vi "Close.vi"(8 "error in (no error)":errorcluster, 11 "Instrument.OxfordVRM in":refnum<class "Instrument.OxfordVRM.lvclass">) -> (0 "error out":errorcluster, 3 "Instrument.OxfordVRM out":refnum<class "Instrument.OxfordVRM.lvclass">)   [LabVIEW 2019, in "Instrument.OxfordVRM.lvclass"]
uses:
  Instrument.OxfordVRM.lvclass
  C:/Program Files (x86)/National Instruments/LabVIEW 2019/user.lib/LevyLab/Instrument Framework/Instrument/Instrument.lvclass
  <userlib>/LevyLab/Instrument Framework/Instrument Types/Cryostat/Instrument.Cryostat.lvclass
  <userlib>/LevyLab/Instrument Framework/Instrument/Instrument.lvclass
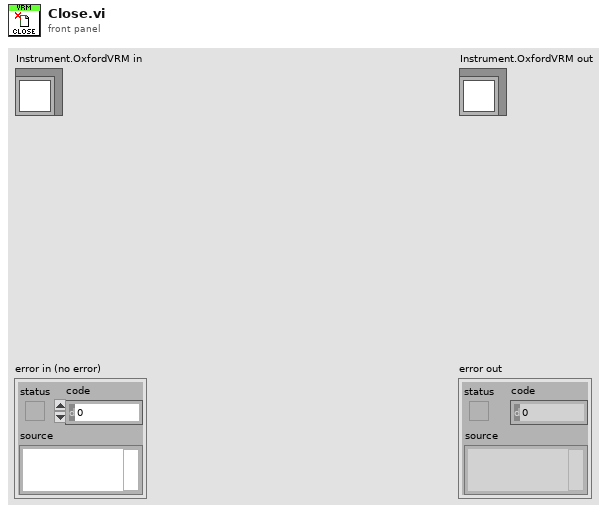
[diagram p1: front panel]
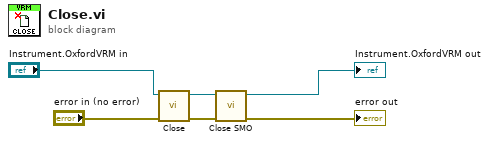
[diagram p0: block diagram]
diagram:
  n1 = call-parent "Close.vi"("error in (no error)"="error in (no error)", "Instrument in"="Instrument.OxfordVRM in") -> ("error out"=w3:errorcluster, "Instrument out"=w4:refnum<class "Instrument.OxfordVRM.lvclass">)  [unwired: 8 in]
  n2 = call <userlib>:"Close SMO.vi"("error in (no error)"=w3, "Instrument in"=w4) -> ("error out"=→"error out":errorcluster, "Instrument out"=→"Instrument.OxfordVRM out":refnum<class "Instrument.OxfordVRM.lvclass">)  [unwired: 8 in]
